vi "Execute.vi"(8 "error in (no error)":errorcluster, 11 "Sell Stock Order in":refnum<class "Sell Stock Order.lvclass">) -> (0 "error out":errorcluster, 3 "Order Out":refnum<class "Order.lvclass">)   [LabVIEW 2019, in "Sell Stock Order.lvclass"]
doc: "Execute the Sell action (Concrete Command) on the Stock Trade (Receiver)"
uses:
  Sell Stock Order.lvclass
  C:/Users/Tiba/Desktop/Command Pattern 2014/Command Pattern 2014/Order/Order.lvclass
  Order/Order.lvclass
  Sell Stock Order.lvclass/Sell Stock Order.ctl
  Stock Trader/Stock Trader.lvclass
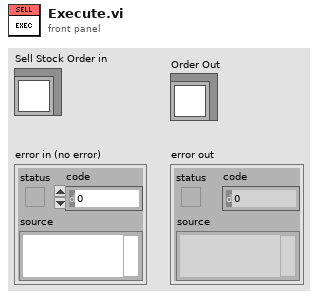
[diagram p1: front panel]
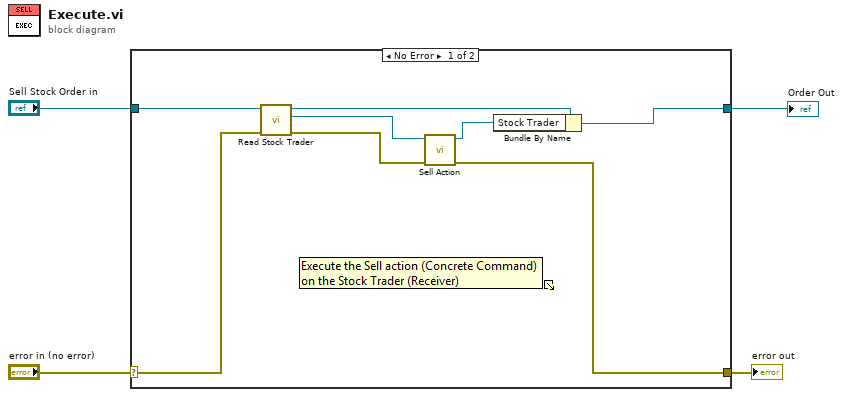
[diagram p0: block diagram]
diagram:
  n1 = case shown="No Error" "error in (no error)" {
    selector: "error in (no error)" -> [w11 w14]
    tunnel: [w9 w14] -> w3
    tunnel: [w7 w13] -> w1
    tunnel: "Sell Stock Order in" -> [w8 w13]
    frame No Error {
      n2 = call-dynamic "Read Stock Trader.vi"("error in (no error)"=w11, "Order in"=w8) -> ("error out"=w10:errorcluster, "Stock Trader"=w12:refnum<class "Stock Trader.lvclass">, "Order out"=w5:refnum<class "Sell Stock Order.lvclass">)  [unwired: 7 in]
      n3 = call "Sell Action.vi"("error in (no error)"=w10, "Stock Trader In"=w12) -> ("error out"=w9:errorcluster, "Stock Trader Out"=w6:refnum<class "Stock Trader.lvclass">)  [unwired: 8 in]
      n4 = Bundle By Name(cluster=w5, "Stock Trader"=w6) -> (w7:refnum<class "Sell Stock Order.lvclass">)
    }
    frame Error {
    }
  }
  "error out" <- w3
  "Order Out" <- w1
